vi "Save Report to File.vi"(0 "report in":refnum<class "NI_Word.lvclass">, 5 "report file path":path, 7 "prompt to replace? (F)":bool, 9 "password (\"\")":string, 11 "error in (no error)":errorcluster) -> (4 "report out":refnum<class "NI_Word.lvclass">, 15 "error out":errorcluster)   [LabVIEW 2020, in "NI_Word.lvclass"]
doc: "Saves an HTML, Word, or Excel report to the file specified in <B>report file path</B>. You cannot use this VI with standard reports."
uses:
  <vilib>/Utility/NIReport.llb/Word/NI_Word.lvclass
  <vilib>/Utility/NIReport.llb/Word/NI_Word.lvclass/NI_Word.ctl
  <vilib>/Utility/NIReport.llb/NI_ReportGenerationCore.lvlib
  <vilib>/addons/_office/NI_ReportGenerationToolkit.lvlib
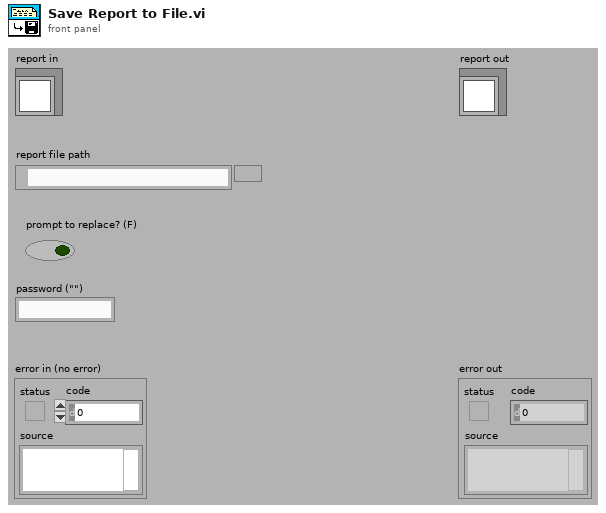
[diagram p1: front panel]
types:
  T1 = enum16{"open", "replace", "create", "open or create", "replace or create", "replace or create with confirmation"}
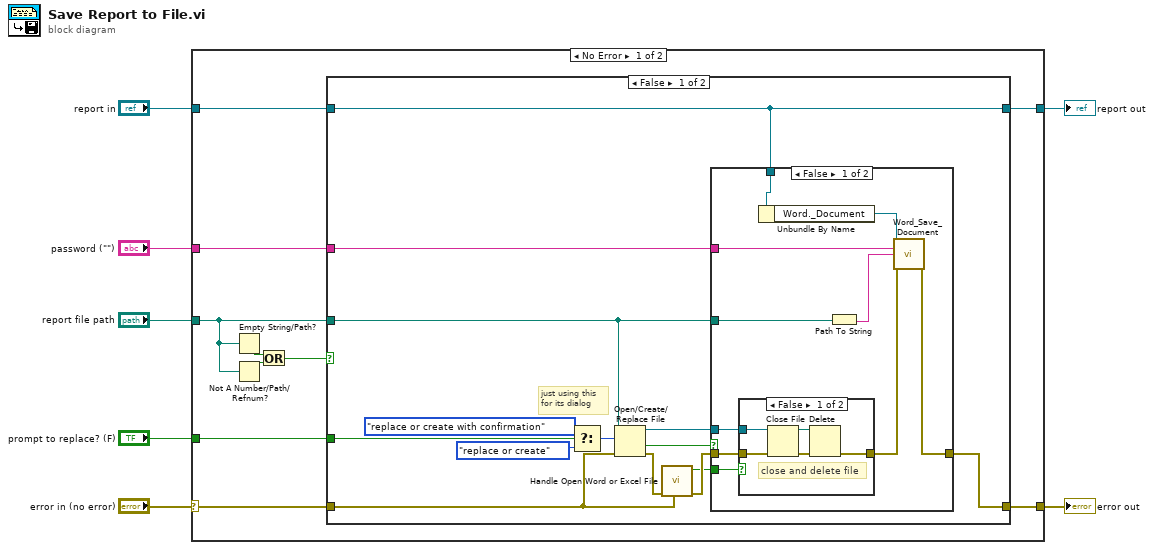
[diagram p0: block diagram]
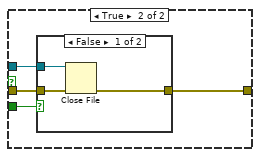
[diagram p3: hidden frame]
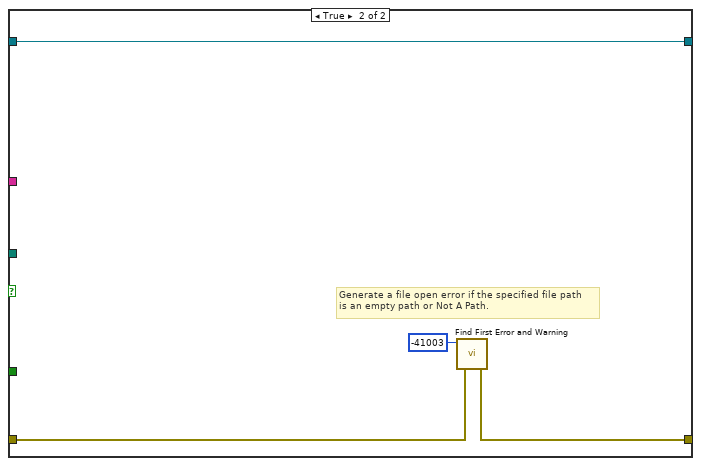
[diagram p5: hidden frame]
diagram:
  n1 = case shown="No Error" "error in (no error)" {
    selector: "error in (no error)" -> [w11 w61]
    tunnel: [w12 w60] -> w5
    tunnel: "report in" -> [w13 w60]
    tunnel: "report file path" -> [w14 _]
    tunnel: [w10 w61] -> w3
    tunnel: "password (\"\")" -> [w9 _]
    tunnel: "prompt to replace? (F)" -> [w8 _]
    frame No Error {
      n2 = Empty String/Path?(string/path=w14) -> (empty?=w16:bool)
      n3 = Not A Number/Path/Refnum?(number/path/refnum=w14) -> (NaN/Path/Refnum?=w15:bool)
      n4 = Or(x=w16, y=w15) -> (x .or. y?=w17:bool)
      n5 = case shown="False" w17 {
        tunnel: [w31 w59] -> w12
        tunnel: w13 -> [w31 w59]
        tunnel: w14 -> [w21 _]
        tunnel: w11 -> [w20 w57]
        tunnel: [w25 w56] -> w10
        tunnel: w9 -> [w30 _]
        tunnel: w8 -> [w22 _]
        frame False {
          # "just using this for its dialog"
          n6 = Select(t=T1."replace or create with confirmation" ("operation (0:open)"), s=w22, f=T1."replace or create" ("operation (0:open)")) -> (s? t:f=w27:T1)
          n7 = Open/Create/Replace File(file path (use dialog)=w21, error in=w20, operation (0:open)=w27) -> (refnum out=w26:refnum<file>, cancelled=w19:bool, error out=w23:errorcluster)  [unwired: 3 out]
          n8 = call <vilib>:"Handle Open Word or Excel File.vi"("previous error"=w20, "file error"=w23) -> ("error out"=w24:errorcluster, "Error 5 or 6?"=w18:bool)  [unwired: 4 in, 4 out]
          n9 = case shown="False" w19 {
            tunnel: w31 -> [w39 _]
            tunnel: w30 -> [w38 _]
            tunnel: w21 -> [w37 _]
            tunnel: w26 -> [w36 w51]
            tunnel: w24 -> [w35 w50]
            tunnel: [w33 w49] -> w25
            tunnel: w18 -> [w32 w48]
            frame False {
              n10 = case shown="False" w32 {
                tunnel: w36 -> [w46 _]
                tunnel: w35 -> [w44 w47]
                tunnel: [w42 w47] -> w34
                frame False {
                  # "close and delete file"
                  n11 = Close File(refnum=w46, error in=w44) -> (path=w45:path, error out=w43:errorcluster)
                  n12 = Delete(path (use dialog)=w45, error in=w43) -> (error out=w42:errorcluster)  [unwired: 5 out]
                }
                frame True {
                }
              }
              n13 = Unbundle By Name(w39) -> ("Word._Document"=w40:refnum<k7>)
              n14 = Path To String(path=w37) -> (string=w41:string)
              n15 = call <vilib>:"Word_Save_Document.vi"("Word._Document"=w40, "password"=w38, "path"=w41, "error in (no error)"=w34) -> ("error out"=w33:errorcluster)  [unwired: 1 in, 10 out]
            }
            frame True {
              n16 = case shown="False" w48 {
                tunnel: w51 -> [w54 _]
                tunnel: w50 -> [w53 w55]
                tunnel: [w52 w55] -> w49
                frame False {
                  n17 = Close File(refnum=w54, error in=w53) -> (error out=w52:errorcluster)  [unwired: 1 out]
                }
                frame True {
                }
              }
            }
          }
        }
        frame True {
          # "Generate a file open error if the specified file path\nis an empty path or Not A Path."
          n18 = call <vilib>:"Find First Error and Warning.vi"("error in (no error)"=w57, "error code"=-41003) -> ("error out"=w56:errorcluster)  [unwired: 1 in, 4 out]
        }
      }
    }
    frame Error {
    }
  }
  "error out" <- w3
  "report out" <- w5
